vi "Store UID Index Value.vi"(8 "error in (no error)":errorcluster, 9 "Assert Count Value":i32, 10 "UID Value":string, 11 "Standard Display Configuration in":refnum<class "Standard Display Configuration.lvclass">) -> (0 "error out":errorcluster, 3 "Standard Display Configuration out":refnum<class "Standard Display Configuration.lvclass">)   [LabVIEW 2016, in "Assert API Components.lvlib" / "Assert Display.lvlib" / "Main Display.lvlib" / "Standard Display Configuration.lvclass"]
doc: "Stores the UID index value in the variant data"
uses:
  Standard Display Configuration.lvclass
  D:/Work/Projects/actor_assert_api/Core/Main Display/Display Configurations/Base Display Configuration.lvclass
  Base Display Configuration.lvclass/Base Display Configuration.ctl
  Base Display Configuration.lvclass
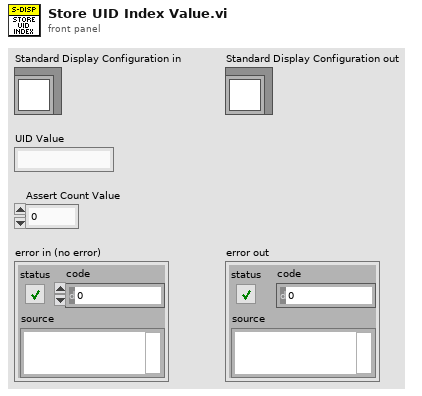
[diagram p1: front panel]
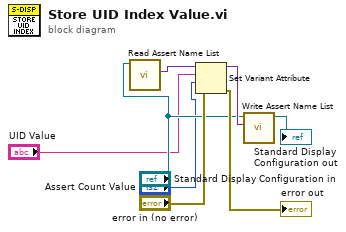
[diagram p0: block diagram]
diagram:
  n1 = call "Read Assert Name List.vi"("Base Display Configuration in"="Standard Display Configuration in") -> ("Assert Name List"=w4:variant)  [unwired: 10 in]
  n2 = Set Variant Attribute(Variant=w4, name="UID Value", value="Assert Count Value", error in="error in (no error)") -> (Variant out=w6:variant, error out=→"error out":errorcluster)  [unwired: 1 out]
  n3 = call "Write Assert Name List.vi"("Assert Name List"=w6, "Base Display Configuration in"="Standard Display Configuration in") -> ("Base Display Configuration out"=→"Standard Display Configuration out":refnum<class "Standard Display Configuration.lvclass">)  [unwired: 9 in]
